vi "I2C_Stop_DAQ.vi"   [LabVIEW 2022 SP3]
panel:
  # "I2C_STOP"
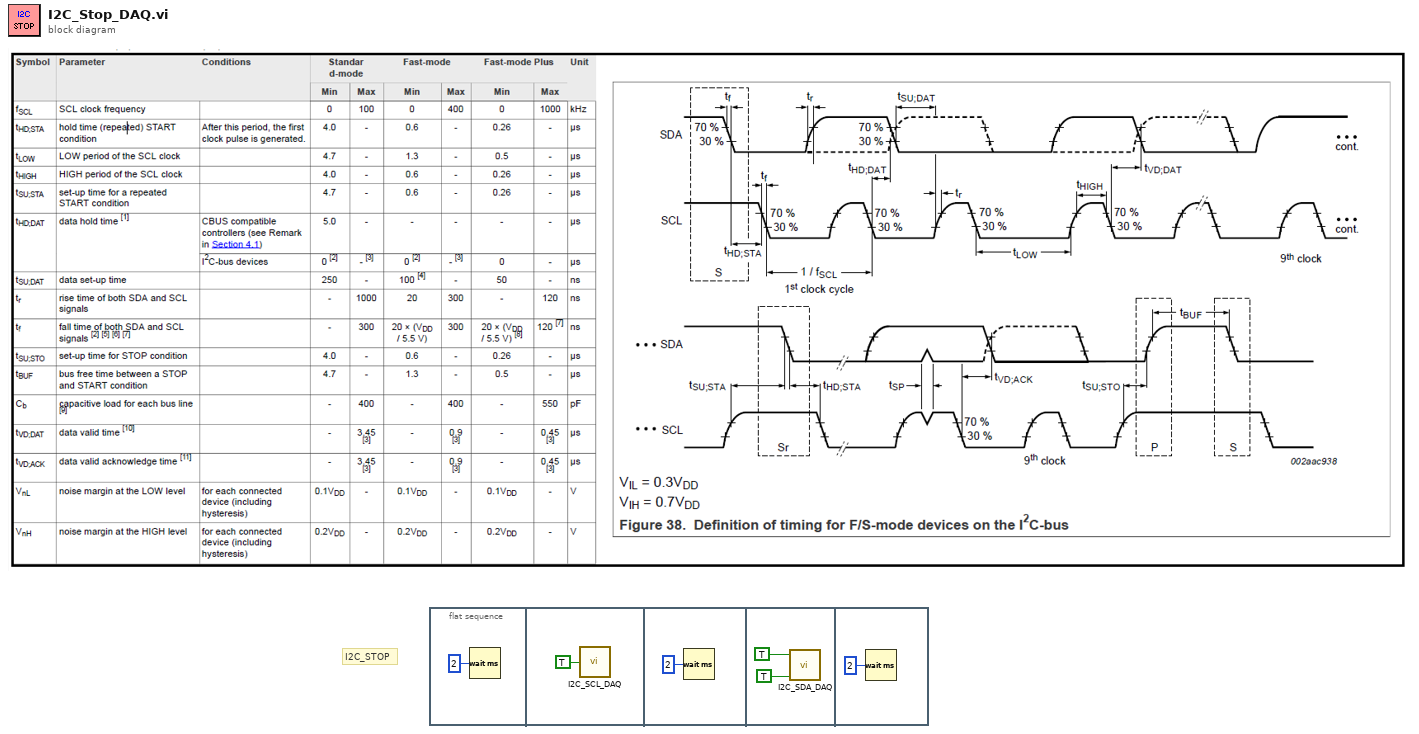
[diagram p0: block diagram]
diagram:
  # "I2C_STOP"
  n1 = flat-sequence {
    frame #0 {
      n2 = Wait (ms)(milliseconds to wait=u32 2) -> ()  [unwired: 1 out]
    }
    frame #1 {
      n3 = call "I2C_SCL_DAQ.vi"("SCL_Data"=TRUE) -> ()  [unwired: 5 in]
    }
    frame #2 {
      n4 = Wait (ms)(milliseconds to wait=u32 2) -> ()  [unwired: 1 out]
    }
    frame #3 {
      n5 = call "I2C_SDA_DAQ.vi"("Tx_or_Rx?"=TRUE, "Tx_Data"=TRUE) -> ()  [unwired: 1 in, 1 out]
    }
    frame #4 {
      n6 = Wait (ms)(milliseconds to wait=u32 2) -> ()  [unwired: 1 out]
    }
  }
